vi "Get User Interface Details.vi"(8 "error in":errorcluster, 11 "measurement plugin service in":refnum<class "Measurement Plugin Service.lvclass">) -> (0 "error out":errorcluster, 2 "user interface details":T1[](array[typedef]), 3 "measurement plugin service out":refnum<class "Measurement Plugin Service.lvclass">)   [LabVIEW 2020, in "MeasurementLink Measurement Server.lvlib" / "Measurement Plugin Service.lvclass"]
uses:
  Measurement Plugin Service.lvclass
  Helpers/TypeDefs/UserInterfaceDetails.ctl
  Helpers/TypeDefs/User Interface Information.ctl
  <vilib>/regexp/Match Regular Expression.xnode
  MeasurementLink Measurement Server.lvlib
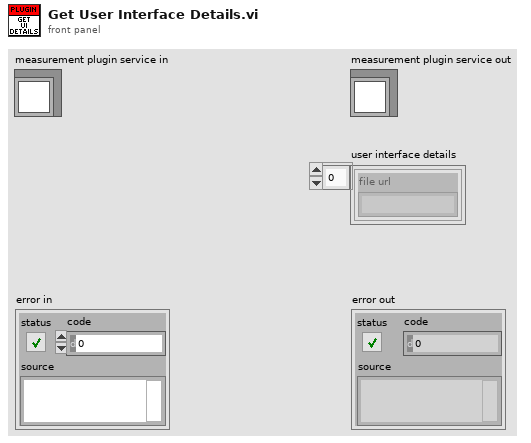
[diagram p1: front panel]
types:
  T1 = typedef "MeasurementLink Measurement Server.lvlib/UserInterfaceDetails.ctl" = cluster{"file url":string}
  T2 = typedef "MeasurementLink Measurement Server.lvlib/User Interface Information.ctl" = cluster{"file":string}
  T3 = typedef "MeasurementLink Measurement Server.lvlib/Measurement Plugin Service.lvclass/Plugin Paths.ctl" = cluster{"get measurement details VI path":path, "get type specializations VI path":path, "get UI details VI path":path, "measurement logic VI path":path, "measurement configuration ctl path":path, "measurement results ctl path":path}
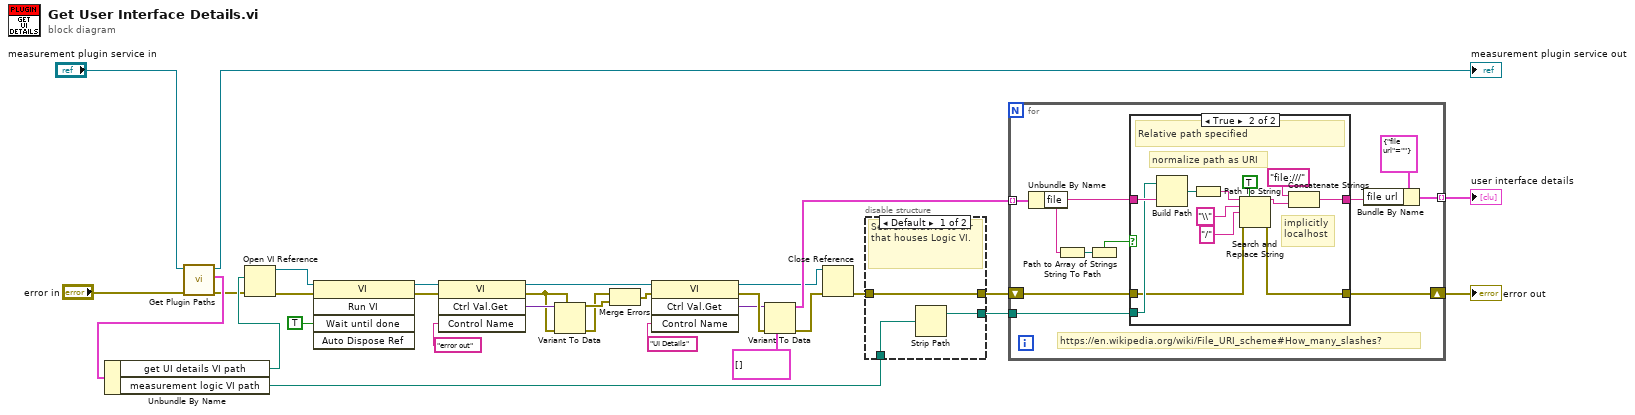
[diagram p0: block diagram]
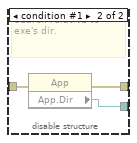
[diagram p2: hidden frame]
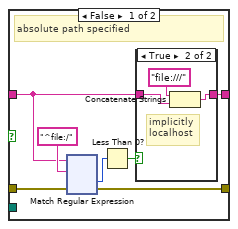
[diagram p3: hidden frame]
diagram:
  n1 = call-dynamic "Get Plugin Paths.vi"("error in"="error in", "measurement plugin service in"="measurement plugin service in") -> ("error out"=w25:errorcluster, "plugin paths"=w27:T3, "measurement plugin service out"=→"measurement plugin service out":refnum<class "Measurement Plugin Service.lvclass">)  [unwired: 7 in]
  n2 = Unbundle By Name(w27) -> ("get UI details VI path"=w26:path, "measurement logic VI path"=w1:path)
  n3 = Open VI Reference(vi path=w26, error in (no error)=w25) -> (vi reference=w8:refnum<vi>, error out=w9:errorcluster)  [unwired: 4 in]
  n4 = invoke class="VI" method="Run VI"(reference=w8, error in=w9, "Wait until done"=TRUE ("Wait Until Done")) -> (reference out=w15:refnum<vi>, error out=w14:errorcluster)  [unwired: 2 in, 3 out]
  n5 = invoke class="VI" method="Ctrl Val.Get"(reference=w15, error in=w14, "Control Name"="error out") -> (reference out=w11:refnum<vi>, error out=w20:errorcluster, "Get Control Value Variant"=w21:variant)  [unwired: 1 in, 1 out]
  n6 = Variant To Data(error in=w20, type=w20, Variant=w21) -> (data=w19:errorcluster, error out=w10:errorcluster)
  n7 = Merge Errors(w10, w19) -> (w13:errorcluster)
  n8 = invoke class="VI" method="Ctrl Val.Get"(reference=w11, error in=w13, "Control Name"="UI Details") -> (reference out=w2:refnum<vi>, error out=w18:errorcluster, "Get Control Value Variant"=w16:variant)  [unwired: 1 in, 1 out]
  n9 = Variant To Data(error in=w18, type=T2[] [], Variant=w16) -> (data=w12:T2[], error out=w4:errorcluster)
  n10 = Close Reference(reference=w2, error in (no error)=w4) -> (error out=w3:errorcluster)
  n11 = disable-structure shown="Default" {
    disable-tunnel: w3 -> [w34 w37]
    disable-tunnel: [w34 w36] -> w5
    disable-tunnel: [w32 w35] -> w6
    disable-tunnel: w1 -> [w33 _]
    frame condition #0 (active) {
      # "Search relative to dir that houses Logic VI."
      n12 = Strip Path(path=w33) -> (stripped path=w32:path)  [unwired: 1 out]
    }
    frame condition #1 {
      # "Search relative to exe's dir."
      n13 = property class="App"(error in=w37) -> (error out=w36:errorcluster, "App.Dir"=w35:path)  [unwired: 1 in, 1 out]
    }
  }
  n14 = for {
    tunnel: w12 -> [w45] mode=indexing
    tunnel: [w46] -> w28 mode=indexing
    shift-right: [w38] -> w7
    shift-left: w5 -> [w39]
    tunnel: w6 -> [w42]
    # "https://en.wikipedia.org/wiki/File_URI_scheme#How_many_slashes?"
    n15 = Unbundle By Name(w45) -> ("file"=w41:string)
    n16 = String To Path(string=w41) -> (path=w44:path)
    n17 = Path to Array of Strings(0:w44) -> (1:w43:bool)  [unwired: 1 out]
    n18 = case shown="True" w43 {
      tunnel: w42 -> [_ w183]
      tunnel: w41 -> [w50 w184]
      tunnel: [w49 w180] -> w40
      tunnel: w39 -> [w53 w174]
      tunnel: [w48 w173] -> w38
      frame False {
        # "absolute path specified"
        n19 = xnode "Match Regular Expression"("input string"=w50, "regular expression"="^file:/", "error in"=w53) -> ("offset past match"=w52:i32, "error out"=w48:errorcluster)  [unwired: 3 in, 3 out]
        n20 = Less Than 0?(x=w52) -> (x < 0?=w51:bool)
        n21 = case shown="True" w51 {
          tunnel: w50 -> [w55 w57]
          tunnel: [w55 w56] -> w49
          frame False {
            # "already uri.\npreserve it"
          }
          frame True {
            # "implicitly\nlocalhost"
            n22 = Concatenate Strings("file:///" ("string"), w57) -> (w56:string)
          }
        }
      }
      frame True {
        # "normalize path as URI"
        # "implicitly\nlocalhost"
        # "Relative path specified"
        n23 = Build Path(base path=w183, name or relative path=w184) -> (appended path=w182:path)
        n24 = Path To String(path=w182) -> (string=w178:string)
        n25 = Search and Replace String(replace all?=TRUE ("replace all? (F)"), input string=w178, search string="\\", replace string="/" ("replace string (\"\")"), error in=w174) -> (result string=w175:string, error out=w173:errorcluster)  [unwired: 3 in, 2 out]
        n26 = Concatenate Strings("file:///" ("string"), w175) -> (w180:string)
      }
    }
    n27 = Bundle By Name(cluster=T1 {"file url"=""} ("UserInterfaceDetails"), "file url"=w40) -> (w46:T1)
  }
  "error out" <- w7
  "user interface details" <- w28
